vi "Fault List 2 Indicators.vi"(10 "Use LBCB Selector":bool, 11 "LBCB Number":T1) -> (0 "Commands":bool, 1 "Forces":bool, 2 "Displacement":bool, 3 "Increments":bool)   [LabVIEW 2013]
uses:
  Data Access Objects/Metadata/LBCB Number.ctl
  Faults List Actions.ctl
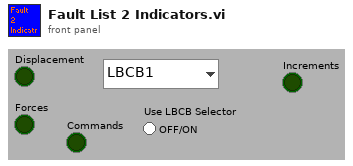
[diagram p1: front panel]
types:
  T1 = typedef "LBCB Number.ctl" = enum16{"LBCB1", "LBCB2"}
  T2 = typedef "Faults List Actions.ctl" = enum16{"Init", "Add", "Remove", "Get List"}
  T3 = typedef "Fault Id.ctl" = cluster{"Fault Type":T4, "LBCB Number":T1, "Index":u32, "Space Type":T5}
  T4 = typedef "Fault Type.ctl" = enum16{"None", "Command", "Displacement", "Force", "Increment"}
  T5 = typedef "Space Type.ctl" = enum16{"Actuator", "Cartesian"}
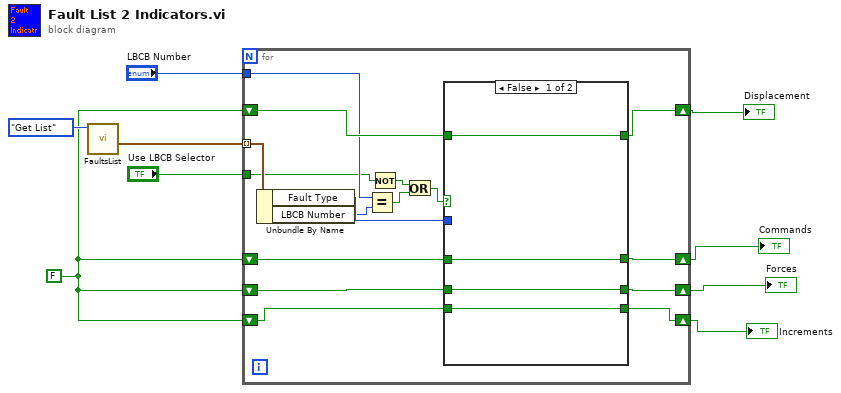
[diagram p0: block diagram]
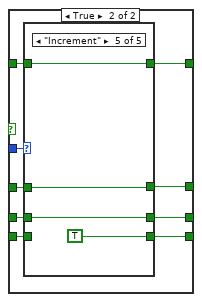
[diagram p2: hidden frame]
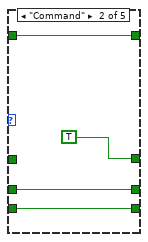
[diagram p4: hidden frame]
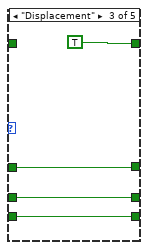
[diagram p5: hidden frame]
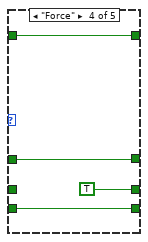
[diagram p6: hidden frame]
diagram:
  w2 = FALSE
  n1 = call "FaultsList.vi"("Limits List Actions"=Faults_List_Actions."Get List") -> ("Fault List"=w8:T3[])  [unwired: 2 in, 8 out]
  n2 = for {
    shift-right: [w23] -> w7
    shift-left: w2 -> [w21]
    shift-right: [w22] -> w6
    shift-left: w2 -> [w20]
    tunnel: w8 -> [w25] mode=indexing
    shift-right: [w19] -> w4
    shift-left: w2 -> [w16]
    tunnel: "LBCB Number" -> [w17]
    tunnel: "Use LBCB Selector" -> [w12]
    shift-right: [w11] -> w1
    shift-left: w2 -> [w10]
    n3 = Unbundle By Name(w25) -> ("Fault Type"=w24:T4, "LBCB Number"=w18:T1)
    n4 = Equal?(x=w17, y=w18) -> (x = y?=w15:bool)
    n5 = Not(x=w12) -> (.not. x?=w13:bool)
    n6 = Or(x=w13, y=w15) -> (x .or. y?=w14:bool)
    n7 = case shown="False" w14 {
      tunnel: w24 -> [_ w38]
      tunnel: [w29 w37] -> w23
      tunnel: [w27 w36] -> w22
      tunnel: w21 -> [w29 w35]
      tunnel: w20 -> [w27 w34]
      tunnel: [w28 w33] -> w19
      tunnel: w16 -> [w28 w32]
      tunnel: [w26 w31] -> w11
      tunnel: w10 -> [w26 w30]
      frame False {
      }
      frame True {
        n8 = case shown="\"Increment\"" w38 {
          tunnel: [w42 w46 TRUE w53 w58] -> w37
          tunnel: [w41 w45 w49 TRUE w55] -> w36
          tunnel: w35 -> [w42 w46 _ w53 w58]
          tunnel: w34 -> [w41 w45 w49 _ w55]
          tunnel: [w40 TRUE w48 w52 w57] -> w33
          tunnel: w32 -> [w40 _ w48 w52 w57]
          tunnel: [w39 w43 w47 w51 TRUE] -> w31
          tunnel: w30 -> [w39 w43 w47 w51 _]
          frame "None" {
          }
          frame "Command" {
          }
          frame "Displacement" {
          }
          frame "Force" {
          }
          frame "Increment" {
          }
        }
      }
    }
  }
  "Displacement" <- w7
  "Forces" <- w6
  "Commands" <- w4
  "Increments" <- w1
